vi "Measurement UI.vi"() -> ()   [LabVIEW 2025, in "Switch Executive Controller UI.lvlib"]
uses:
  Switch Executive Controller UI.lvlib
  UI Data.ctl
  <vilib>/SwitchExecutive/nise.llb/niSE SessionRefnum.ctl
panel:
  out "Last Route":string
  out "Last SE Device":string
  in  "DUT Pin":string
  in  "DUT Route":bool
  in  "Route Specification":string
  in  "Routes":string[](tree)
  in  "Operation":T1(ring)
  in  "Refresh":bool
  in  "Switch Executive Virtual Device":string(combo) caption="Pin name"
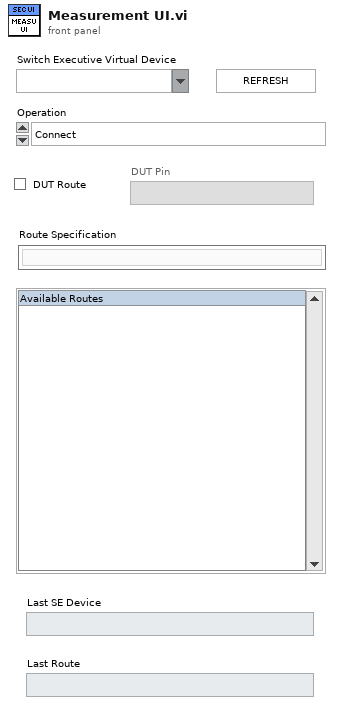
[diagram p1: front panel]
types:
  T1 = enum32{"Connect", "Disconnect", "Disconnect All"}
  T2 = typedef "Switch Executive Controller UI.lvlib/UI Data.ctl" = cluster{"NISE Session":T3, "Session Open?":bool, "SE Virtual Device":string}
  T3 = typedef "niSE SessionRefnum.ctl" = refnum<k1>
  T4 = enum8{"Enabled", "Disabled", "Disabled and Grayed Out"}
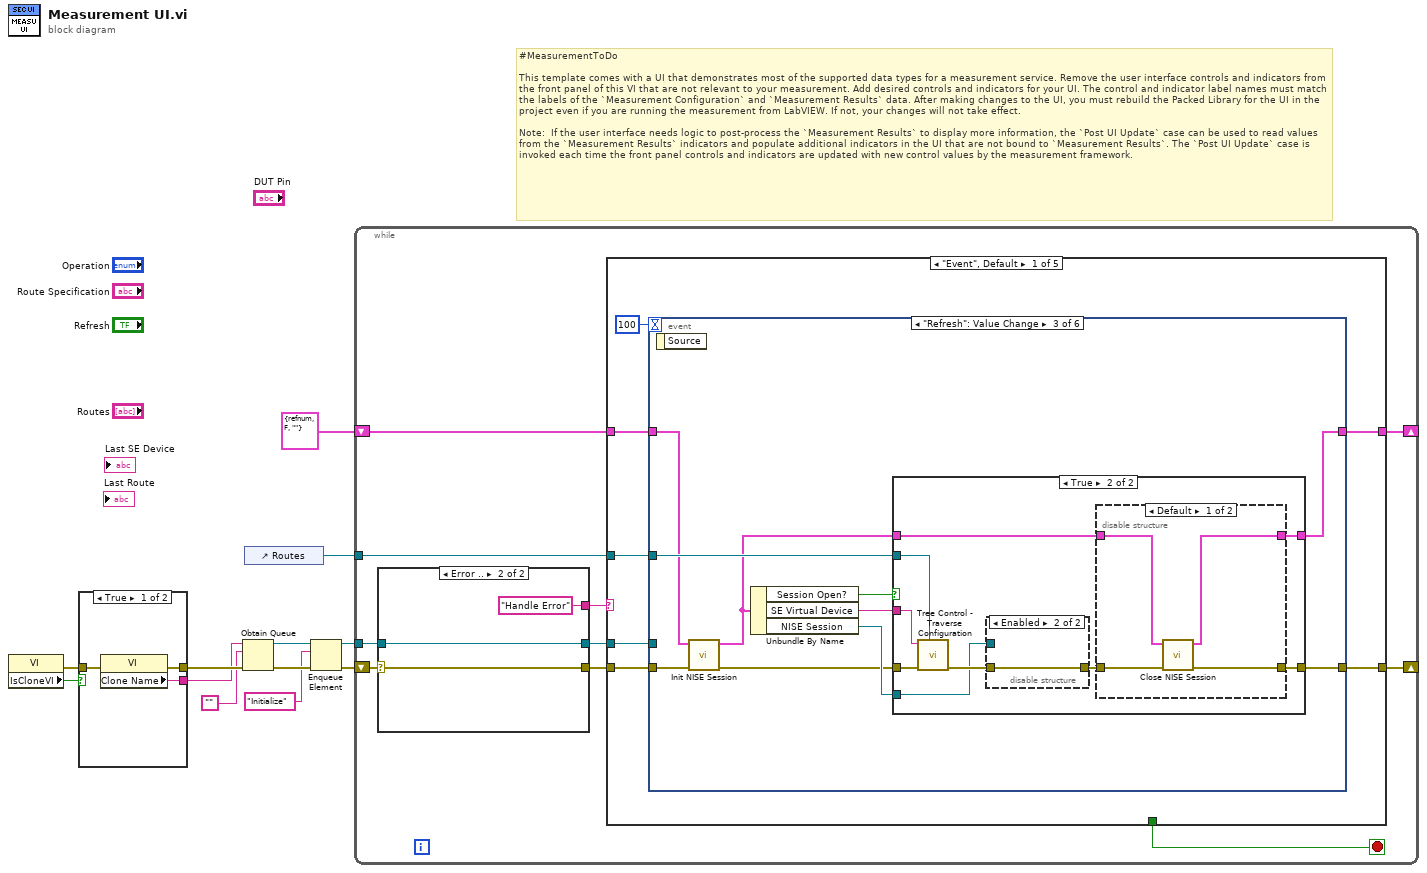
[diagram p0: block diagram]
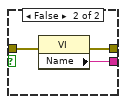
[diagram p2: hidden frame]
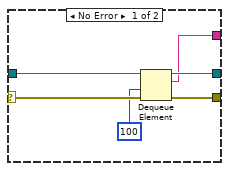
[diagram p3: hidden frame]
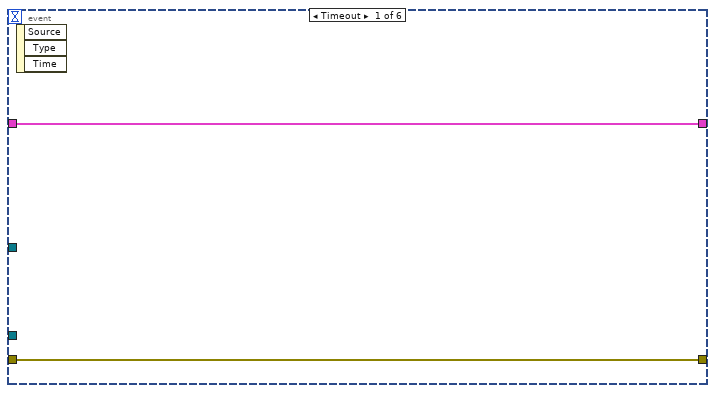
[diagram p4: hidden frame]
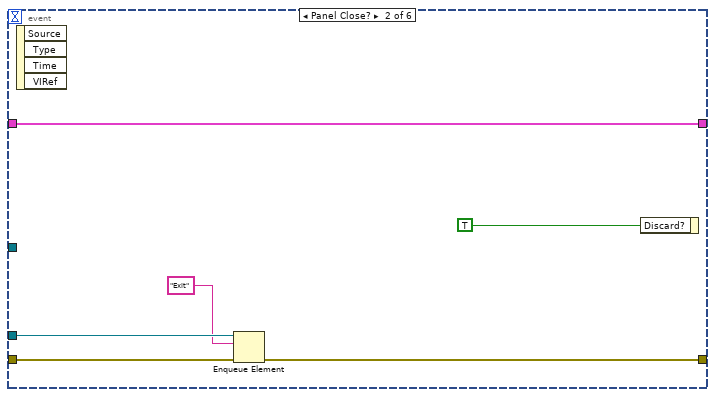
[diagram p5: hidden frame]
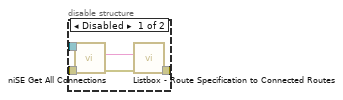
[diagram p7: hidden frame]
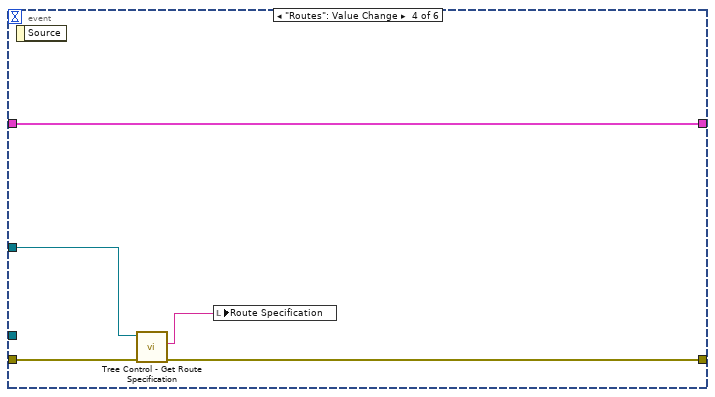
[diagram p9: hidden frame]
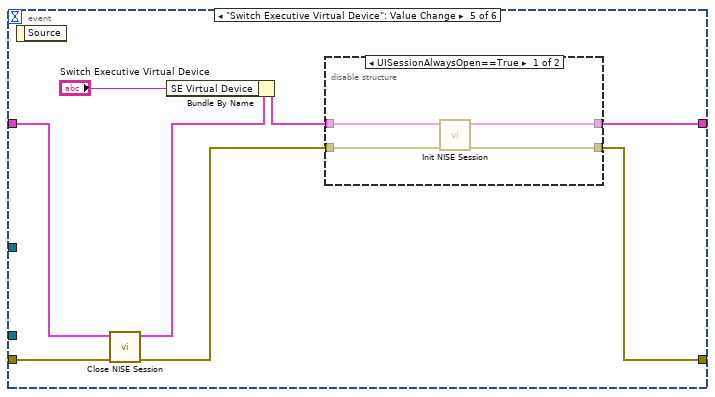
[diagram p10: hidden frame]
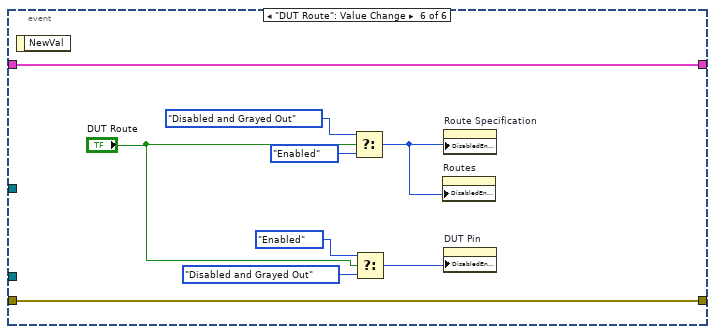
[diagram p12: hidden frame]
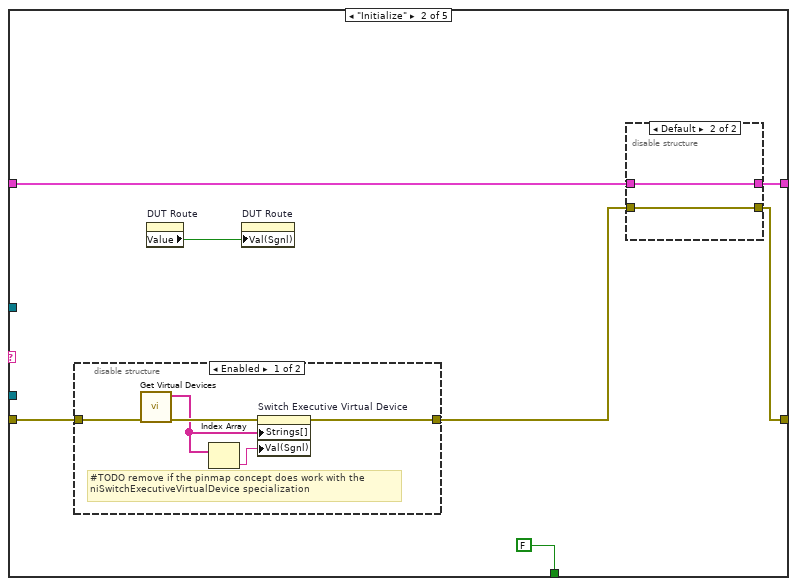
[diagram p13: hidden frame]
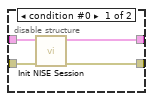
[diagram p14: hidden frame]
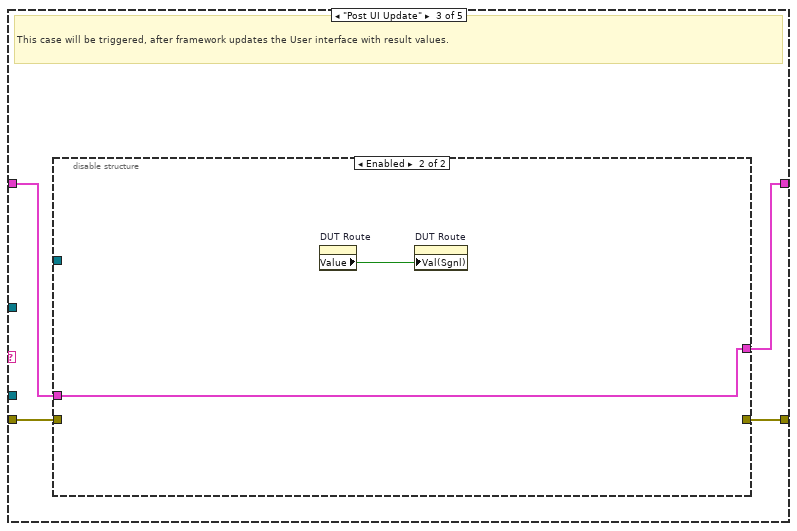
[diagram p16: hidden frame]
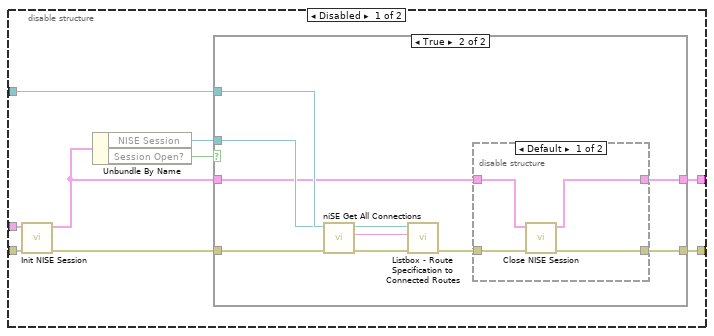
[diagram p17: hidden frame]
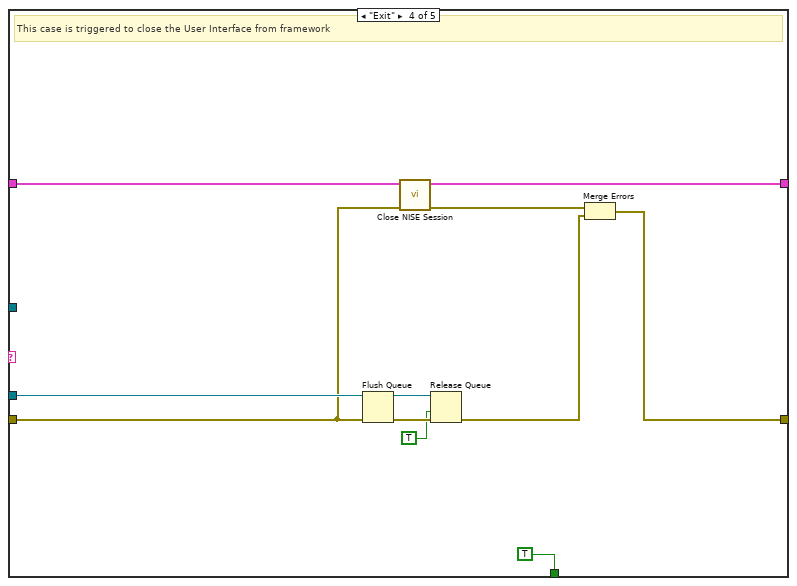
[diagram p20: hidden frame]
diagram:
  # "#MeasurementToDo  \n\nThis template comes with a UI that demonstrates most of the supported data types for a measurement service. Remove the user interface controls and indicators from the front panel of this VI that are not relevant to your measurement. Add desired controls and indicators for your UI. The control and indicator label names must match the labels of the `Measurement Configuration` and `Measurement Results` data. After making changes to the UI, you must rebuild the Packed Library for the UI in the project even if you are running the measurement from LabVIEW. If not, your changes will not take effect.\n\nNote:  If the user interface needs logic to post-process the `Measurement Results` to display more information, the `Post UI Update` case can be used to read values from the `Measurement Results` indicators and populate additional indicators in the UI that are not bound to `Measurement Results`. The `Post UI Update` case is invoked each time the front panel controls and indicators are updated with new control values by the measurement framework."
  n1 = property class="VI"() -> (error out=w3:errorcluster, "IsCloneVI"=w4:bool)  [unwired: 2 in, 1 out]
  n2 = case shown="True" w4 {
    tunnel: [w15 w18] -> w12
    tunnel: [w14 w17] -> w11
    tunnel: w3 -> [w13 w16]
    frame True {
      n3 = property class="VI"(error in=w13) -> (error out=w15:errorcluster, "Clone Name"=w14:string)  [unwired: 1 in, 1 out]
    }
    frame False {
      n4 = property class="VI"(error in=w16) -> (error out=w18:errorcluster, "Name"=w17:string)  [unwired: 1 in, 1 out]
    }
  }
  n5 = Obtain Queue(name (unnamed)=w11, element data type="", error in (no error)=w12) -> (queue out=w8:refnum<queue>, error out=w10:errorcluster)  [unwired: 2 in, 1 out]
  n6 = control-ref of="Routes"() -> (w2:refnum<vi>)
  n7 = Enqueue Element(queue=w8, element="Initialize", error in (no error)=w10) -> (queue out=w7:refnum<queue>, error out=w9:errorcluster)  [unwired: 1 in, 1 out]
  n8 = while {
    shift-right: [w23] -> _
    shift-left: w9 -> [w28]
    tunnel: w7 -> [w26]
    tunnel: w2 -> [w21]
    shift-right: [w19] -> _
    shift-left: T2 {"NISE Session"=refnum, "Session Open?"=FALSE, "SE Virtual Device"=""} ("UI Data") -> [w20]
    stop <- w22 stop-if-true
    n9 = case shown="Error .." w28 {
      selector: w28 -> [w34 w37]
      tunnel: [w33 w37] -> w27
      tunnel: w26 -> [w32 w36]
      tunnel: [w31 w36] -> w25
      tunnel: [w30 "Handle Error"] -> w24
      frame No Error {
        n10 = Dequeue Element(queue=w32, timeout in ms (-1)=100, error in (no error)=w34) -> (queue out=w31:refnum<queue>, element=w30:string, error out=w33:errorcluster)  [unwired: 1 out]
      }
      frame Error {
      }
    }
    n11 = case shown="\"Event\", Default" w24 {
      tunnel: w27 -> [w43 w119 w134 w167 w179]
      tunnel: w25 -> [w41 _ _ w174 _]
      tunnel: [w44 w118 w136 w166 w177] -> w23
      tunnel: [_ FALSE _ TRUE _] -> w22
      tunnel: w21 -> [w40 _ _ _ _]
      tunnel: w20 -> [w39 w116 w135 w170 w176]
      tunnel: [w38 w117 w133 w169 w176] -> w19
      frame "Event", Default {
        n12 = event shown="[2] \"Refresh\": Value Change" {
          selector: _ -> [_ _ _ _ _ _]
          dyn-events: _ -> [_ _ _ _ _ _]
          timeout: 100 -> [_ _ _ _ _ _]
          tunnel: [w46 w50 w62 w87 w97 w112] -> w44
          tunnel: w43 -> [w46 w51 w60 w89 w95 w112]
          tunnel: w41 -> [_ w49 _ _ _ _]
          tunnel: w40 -> [_ _ w61 w90 _ _]
          tunnel: w39 -> [w45 w47 w58 w86 w96 w113]
          tunnel: [w45 w47 w59 w86 w98 w113] -> w38
          event Timeout {
            n13 = event-data() -> ()  [unwired: 1 in, 3 out]
          }
          event Panel Close? {
            n14 = event-data() -> ()  [unwired: 1 in, 4 out]
            n15 = Enqueue Element(queue=w49, element="Exit", error in (no error)=w51) -> (error out=w50:errorcluster)  [unwired: 1 in, 2 out]
            n16 = event-data("Discard?"=TRUE) -> ()  [unwired: 1 in, 1 out]
          }
          event "Refresh": Value Change {
            n17 = event-data() -> ()  [unwired: 1 in, 1 out]
            n18 = call "Init NISE Session.vi"("error in (no error)"=w60, "UI Data in"=w58) -> ("error out"=w54:errorcluster, "UI Data out"=w53:T2)  [unwired: 8 in]
            n19 = Unbundle By Name(w53) -> ("Session Open?"=w55:bool, "SE Virtual Device"=w57:string, "NISE Session"=w56:T3)
            n20 = case shown="True" w55 {
              tunnel: w54 -> [w64 w73]
              tunnel: w61 -> [_ w71]
              tunnel: [w64 w67] -> w62
              tunnel: w56 -> [_ w69]
              tunnel: w57 -> [_ w72]
              tunnel: w53 -> [w63 w66]
              tunnel: [w63 w65] -> w59
              frame False {
              }
              frame True {
                n21 = call "Tree Control - Traverse Configuration.vi"("tree refnum"=w71, "error in (no error)"=w73, "virtual device"=w72) -> ("error out"=w70:errorcluster)  [unwired: 7 in, 1 out]
                n22 = disable-structure shown="Enabled" {
                  disable-tunnel: w70 -> [w77 w79]
                  disable-tunnel: w69 -> [w75 _]
                  disable-tunnel: [w74 w79] -> w68
                  frame Disabled {
                    n23 = call <vilib>:"niSE Get All Connections.vi"("error in (no error)"=w77, "NISE Session (in)"=w75) -> ("error out"=w76:errorcluster, "Route Specification"=w78:string)  [unwired: 3 in, 1 out]
                    n24 = call "Listbox - Route Specification to Connected Routes.vi"("error in (no error)"=w76, "route specification"=w78) -> ("error out"=w74:errorcluster)  [unwired: 8 in, 1 out]
                  }
                  frame Enabled {
                  }
                }
                n25 = disable-structure shown="Default" {
                  disable-tunnel: w68 -> [w83 w84]
                  disable-tunnel: [w82 w84] -> w67
                  disable-tunnel: w66 -> [w81 w85]
                  disable-tunnel: [w80 w85] -> w65
                  frame condition #0 (active) {
                    n26 = call "Close NISE Session.vi"("error in (no error)"=w83, "UI Data in"=w81) -> ("error out"=w82:errorcluster, "UI Data out"=w80:T2)  [unwired: 8 in]
                  }
                  frame condition #1 {
                  }
                }
              }
            }
          }
          event "Routes": Value Change {
            n27 = event-data() -> ()  [unwired: 1 in, 1 out]
            n28 = call "Tree Control - Get Route Specification.vi"("error in (no error)"=w89, "tree refnum"=w90) -> ("error out"=w87:errorcluster, "route specification"=w88:string)  [unwired: 7 in, 1 out]
            n29 = local write "Route Specification"(w88) -> ()
          }
          event "Switch Executive Virtual Device": Value Change {
            n30 = event-data() -> ()  [unwired: 1 in, 1 out]
            n31 = call "Close NISE Session.vi"("error in (no error)"=w95, "UI Data in"=w96) -> ("error out"=w93:errorcluster, "UI Data out"=w94:T2)  [unwired: 8 in]
            n32 = Bundle By Name(cluster=w94, "SE Virtual Device"="Switch Executive Virtual Device") -> (w92:T2)
            n33 = disable-structure shown="UISessionAlwaysOpen==True" {
              disable-tunnel: [w102 w104] -> w98
              disable-tunnel: [w101 w103] -> w97
              disable-tunnel: w93 -> [w100 w103]
              disable-tunnel: w92 -> [w99 w104]
              frame condition #0 {
                n34 = call "Init NISE Session.vi"("error in (no error)"=w100, "UI Data in"=w99) -> ("error out"=w101:errorcluster, "UI Data out"=w102:T2)  [unwired: 8 in]
              }
              frame condition #1 (active) {
              }
            }
          }
          event "DUT Route": Value Change {
            n35 = event-data() -> ()  [unwired: 1 in, 1 out]
            n36 = Select(t=T4."Disabled and Grayed Out" ("Disabled"), s="DUT Route", f=T4."Enabled") -> (s? t:f=w109:T4)
            n37 = Select(t=T4."Enabled" ("Disabled"), s="DUT Route", f=T4."Disabled and Grayed Out") -> (s? t:f=w105:T4)
            n38 = property on="Routes" class="Tree (strict)"("DisabledEnum"=w109) -> ()  [unwired: 2 in, 2 out]
            n39 = property on="Route Specification" class="Str"("DisabledEnum"=w109) -> ()  [unwired: 2 in, 2 out]
            n40 = property on="DUT Pin" class="Str"("DisabledEnum"=w105) -> ()  [unwired: 2 in, 2 out]
          }
        }
      }
      frame "Initialize" {
        n41 = disable-structure shown="Enabled" {
          disable-tunnel: w119 -> [w131 w132]
          disable-tunnel: [w129 w132] -> w115
          frame Enabled {
            # "#TODO remove if the pinmap concept does work with the \nniSwitchExecutiveVirtualDevice specialization"
            n42 = call "Get Virtual Devices.vi"("error in"=w131) -> ("error out"=w130:errorcluster, "Virtual Devices"=w128:string[])  [unwired: 9 in]
            n43 = Index Array(array=w128) -> (element=w127:string)  [unwired: 1 in]
            n44 = property on="Switch Executive Virtual Device" class="CmbBox"(error in=w130, "Strings[]"=w128, "Val(Sgnl)"=w127) -> (error out=w129:errorcluster)  [unwired: 1 in, 1 out]
          }
          frame Disabled {
          }
        }
        n45 = property on="DUT Route" class="Bool (strict)"() -> ("Value"=w114:bool)  [unwired: 2 in, 2 out]
        n46 = property on="DUT Route" class="Bool (strict)"("Val(Sgnl)"=w114) -> ()  [unwired: 2 in, 2 out]
        n47 = disable-structure shown="Default" {
          disable-tunnel: w115 -> [w124 w125]
          disable-tunnel: [w123 w125] -> w118
          disable-tunnel: [w122 w126] -> w117
          disable-tunnel: w116 -> [w121 w126]
          frame condition #0 {
            n48 = call "Init NISE Session.vi"("error in (no error)"=w124, "UI Data in"=w121) -> ("error out"=w123:errorcluster, "UI Data out"=w122:T2)  [unwired: 8 in]
          }
          frame condition #1 (active) {
          }
        }
      }
      frame "Post UI Update" {
        # "This case will be triggered, after framework updates the User interface with result values."
        n49 = disable-structure shown="Enabled" {
          disable-tunnel: [w145 _] -> w136
          disable-tunnel: _ -> [w144 _]
          disable-tunnel: w135 -> [w141 w164]
          disable-tunnel: w134 -> [w139 _]
          disable-tunnel: [w137 w164] -> w133
          frame Disabled {
            n50 = call "Init NISE Session.vi"("error in (no error)"=w139, "UI Data in"=w141) -> ("error out"=w140:errorcluster, "UI Data out"=w138:T2)  [unwired: 8 in]
            n51 = Unbundle By Name(w138) -> ("NISE Session"=w142:T3, "Session Open?"=w143:bool)
            n52 = case shown="True" w143 {
              tunnel: w140 -> [w147 w155]
              tunnel: w144 -> [_ w153]
              tunnel: [w147 w150] -> w145
              tunnel: w142 -> [_ w152]
              tunnel: w138 -> [w146 w149]
              tunnel: [w146 w148] -> w137
              frame False {
              }
              frame True {
                n53 = call <vilib>:"niSE Get All Connections.vi"("error in (no error)"=w155, "NISE Session (in)"=w152) -> ("error out"=w154:errorcluster, "Route Specification"=w156:string)  [unwired: 3 in, 1 out]
                n54 = call "Listbox - Route Specification to Connected Routes.vi"("error in (no error)"=w154, "route specification"=w156, "listbox reference"=w153) -> ("error out"=w151:errorcluster)  [unwired: 7 in, 1 out]
                n55 = disable-structure shown="Default" {
                  disable-tunnel: w151 -> [w160 w161]
                  disable-tunnel: [w159 w161] -> w150
                  disable-tunnel: w149 -> [w158 w162]
                  disable-tunnel: [w157 w162] -> w148
                  frame condition #0 (active) {
                    n56 = call "Close NISE Session.vi"("error in (no error)"=w160, "UI Data in"=w158) -> ("error out"=w159:errorcluster, "UI Data out"=w157:T2)  [unwired: 8 in]
                  }
                  frame condition #1 {
                  }
                }
              }
            }
          }
          frame Enabled {
            n57 = property on="DUT Route" class="Bool (strict)"() -> ("Value"=w163:bool)  [unwired: 2 in, 2 out]
            n58 = property on="DUT Route" class="Bool (strict)"("Val(Sgnl)"=w163) -> ()  [unwired: 2 in, 2 out]
          }
        }
      }
      frame "Exit" {
        # "This case is triggered to close the User Interface from framework"
        n59 = Flush Queue(queue=w174, error in (no error)=w167) -> (queue out=w173:refnum<queue>, error out=w172:errorcluster)  [unwired: 1 out]
        n60 = call "Close NISE Session.vi"("error in (no error)"=w167, "UI Data in"=w170) -> ("error out"=w168:errorcluster, "UI Data out"=w169:T2)  [unwired: 8 in]
        n61 = Release Queue(queue=w173, force destroy? (F)=TRUE, error in (no error)=w172) -> (error out=w165:errorcluster)  [unwired: 2 out]
        n62 = Merge Errors(w168, w165) -> (w166:errorcluster)
      }
      frame "Handle Error" {
        n63 = call <vilib>:"Simple Error Handler.vi"("error in (no error)"=w179) -> ("error out"=w178:errorcluster)  [unwired: 4 in, 4 out]
        n64 = call <vilib>:"Clear Errors.vi"("error in (no error)"=w178) -> ("error out"=w177:errorcluster)  [unwired: 5 in, 1 out]
      }
    }
  }
